vi "Open Project References.vi"(0 "NI Build Specification":refnum<class "NI Build Specification_LV.lvclass">, 11 "error in (no error)":errorcluster) -> (4 "NI Build Specification":refnum<class "NI Build Specification_LV.lvclass">, 15 "error out":errorcluster)   [LabVIEW 2017, in "CL_G3_VIComponentBuilder.lvlib" / "NI Build Specification_LV.lvclass"]
doc: "Opens project references for this build spec and all sub build specs."
uses:
  NI Build Specification_LV.lvclass
  C:/builds/Component BuilderBT/SrcDist/Exports/Exports/Export.lvclass
  Exports/Export.lvclass/Export.ctl
  NI Build Specification_LV.lvclass/NI Build Specification_LV.ctl
  Exports/Accessors/Write Exported Build Specification Path.vi
  Exports/Accessors/Read Exported Build Specification Path.vi
  Accessors/Read Export's Build Spec Name.vi
  Accessors/Read Target Name Containing Build Specs to Build.vi
  Accessors/Read LabVIEW Project SubBuild Spec Order.vi
  Accessors/Write Project Reference.vi
  Accessors/Write Build Spec Ref.vi
  Accessors/Write TargetRef Containting Build Spec.vi
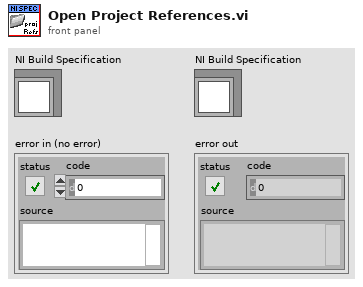
[diagram p1: front panel]
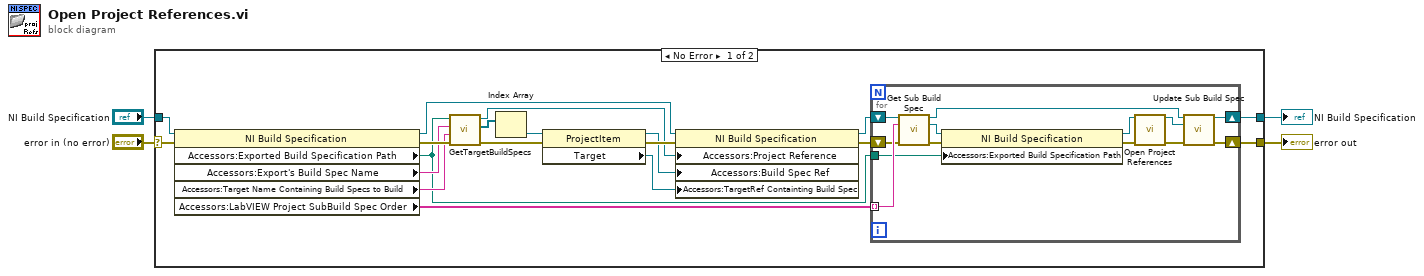
[diagram p0: block diagram]
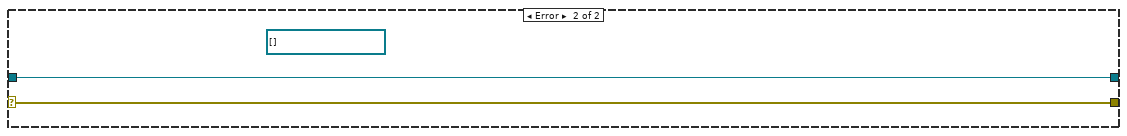
[diagram p2: hidden frame]
diagram:
  n1 = case shown="No Error" "error in (no error)" {
    selector: "error in (no error)" -> [w22 w38]
    tunnel: [w9 w38] -> w3
    tunnel: "NI Build Specification" -> [w23 w37]
    tunnel: [w8 w37] -> w1
    frame No Error {
      n2 = property class="NI Build Specification"(reference=w23, error in=w22) -> (reference out=w20:refnum<class "NI Build Specification_LV.lvclass">, error out=w21:errorcluster, "Accessors:Exported Build Specification Path"=w5:path, "Accessors:Export's Build Spec Name"=w19:string, "Accessors:Target Name Containing Build Specs to Build"=w18:string, "Accessors:LabVIEW Project SubBuild Spec Order"=w14:string[])
      n3 = call <vilib>:"GetTargetBuildSpecs.vi"("error in (no error)"=w21, "Name of target (My Computer)"=w18, "Name of build specification (if empty: get all)"=w19, "Path to project"=w5) -> ("error out"=w16:errorcluster, "buildspec refs"=w17:refnum<vi>[], "project ref"=w6:refnum<vi>)  [unwired: 5 in]
      n4 = Index Array(array=w17) -> (element=w12:refnum<vi>)  [unwired: 1 in]
      n5 = property class="ProjectItem"(reference=w12, error in=w16) -> (reference out=w7:refnum<vi>, error out=w15:errorcluster, "Target"=w11:refnum<vi>)
      n6 = property class="NI Build Specification"(reference=w20, error in=w15, "Accessors:Project Reference"=w6, "Accessors:Build Spec Ref"=w7, "Accessors:TargetRef Containting Build Spec"=w11) -> (reference out=w13:refnum<class "NI Build Specification_LV.lvclass">, error out=w10:errorcluster)
      n7 = for {
        tunnel: w14 -> [w35] mode=indexing
        shift-right: [w32] -> w9
        shift-left: w10 -> [w33]
        shift-right: [w31] -> w8
        shift-left: w13 -> [w36]
        tunnel: w5 -> [w24]
        n8 = call "Get Sub Build Spec.vi"("NI Build Specification in"=w36, "Sub Build Spec Name"=w35, "error in (no error)"=w33) -> ("NI Build Specification out"=w34:refnum<class "NI Build Specification_LV.lvclass">, "Sub Build Spec"=w30:refnum<class "NI Build Specification_LV.lvclass">, "error out"=w26:errorcluster)  [unwired: 9 in, 1 out]
        n9 = property class="NI Build Specification"(reference=w30, error in=w26, "Accessors:Exported Build Specification Path"=w24) -> (reference out=w27:refnum<class "NI Build Specification_LV.lvclass">, error out=w25:errorcluster)
        n10 = call-dynamic "Open Project References.vi"("NI Build Specification"=w27, "error in (no error)"=w25) -> ("NI Build Specification"=w29:refnum<class "NI Build Specification_LV.lvclass">, "error out"=w28:errorcluster)  [unwired: 12 in]
        n11 = call "Update Sub Build Spec.vi"("NI Build Specification in"=w34, "Sub Build Spec"=w29, "error in (no error)"=w28) -> ("NI Build Specification out"=w31:refnum<class "NI Build Specification_LV.lvclass">, "error out"=w32:errorcluster)  [unwired: 11 in]
      }
    }
    frame Error {
      (unwired) refnum<vi>[] []
    }
  }
  "error out" <- w3
  "NI Build Specification" <- w1
